vi "ROI entry-Clear ROI overlay.vi"(8 "error in (no error)":errorcluster) -> (0 "error out":errorcluster, 3 "Image Out":T1)   [LabVIEW 2020]
uses:
  <vilib>/vision/Image Controls.llb/IMAQ Image.ctl
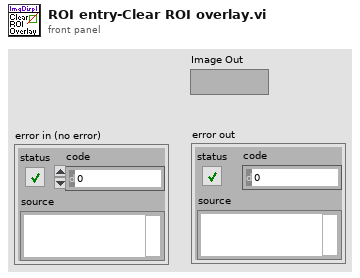
[diagram p1: front panel]
types:
  T1 = typedef "IMAQ Image.ctl" = refnum<image>
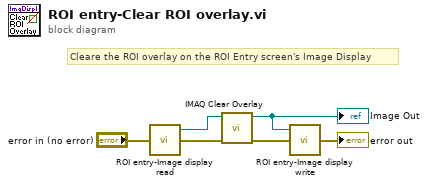
[diagram p0: block diagram]
diagram:
  # "Cleare the ROI overlay on the ROI Entry screen's Image Display"
  n1 = call "ROI entry-Image display read.vi"("error in (no error)"="error in (no error)") -> ("error out"=w4:errorcluster, "CurrentImage"=w6:T1)  [unwired: 3 in]
  n2 = call "IMAQ Clear Overlay"("error in (no error)"=w4, "Image"=w6) -> ("error out"=w3:errorcluster, "Image Out"=w5:T1)  [unwired: 8 in]
  "Image Out" <- w5
  n3 = call "ROI entry-Image display write.vi"("error in (no error)"=w3, "Value"=w5) -> ("error out"=→"error out":errorcluster)  [unwired: 3 in]
